vi "AddMenberToRankingList.vi"(2 "Arr引用句柄":refnum<vi>, 3 "玩家信息":T1, 4 "File Path Control":path) -> ()   [LabVIEW 2019]
uses:
  ctl/InfoOfPlayer.ctl
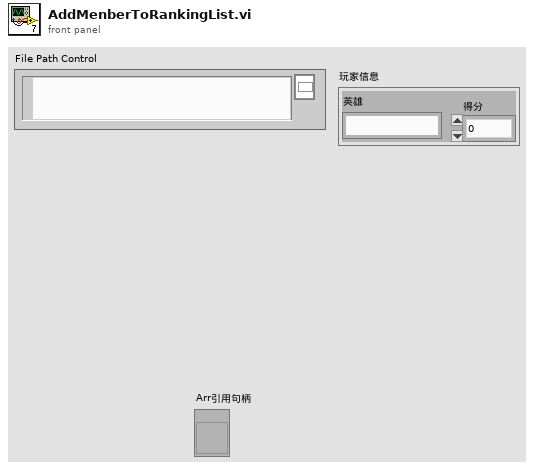
[diagram p1: front panel]
types:
  T1 = typedef "InfoOfPlayer.ctl" = cluster{"得分":i32, "英雄":string}
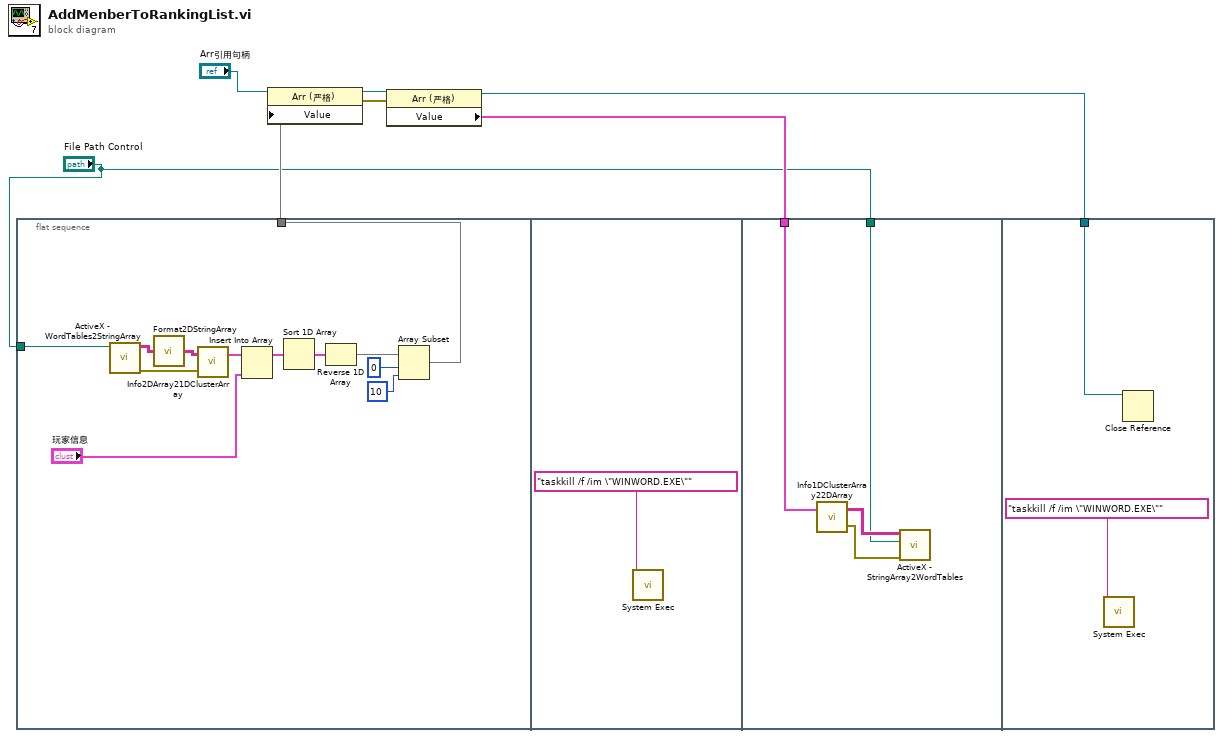
[diagram p0: block diagram]
diagram:
  n1 = flat-sequence {
    tunnel: "File Path Control" -> [w10]
    tunnel: [w8] -> w6
    tunnel: w3 -> [w22]
    tunnel: "File Path Control" -> [w21]
    tunnel: w1 -> [w25]
    frame #0 {
      n2 = call "ActiveX - WordTables2StringArray.vi"("File Path Control"=w10) -> ("Error Out"=w19:errorcluster, "Array"=w11:string[][])  [unwired: 7 in, 2 out]
      n3 = call "Format2DStringArray.vi"("待格式化2D数组"=w11) -> ("格式化2D数组"=w12:string[][])
      n4 = call "Info2DArray21DClusterArray.vi"("error in (no error)"=w19, "2DStringArray"=w12) -> ("1DClusterArray"=w18:T1[])  [unwired: 1 out]
      n5 = Insert Into Array(array=w18, new element="玩家信息") -> (w17:T1[])  [unwired: 1 in]
      n6 = Sort 1D Array(array=w17) -> (sorted array=w14:T1[])
      n7 = Reverse 1D Array(array=w14) -> (reversed array=w13:T1[])
      n8 = Array Subset(array=w13, index=0 ("索引"), length=10 ("长度")) -> (w8:T1[])
    }
    frame #1 {
      n9 = call <vilib>:"System Exec.vi"("command line"="taskkill /f /im \"WINWORD.EXE\"") -> ()  [unwired: 7 in, 4 out]
    }
    frame #2 {
      n10 = call "Info1DClusterArray22DArray.vi"("1D ClusterArray"=w22) -> ("error out"=w24:errorcluster, "2D StringArray"=w23:string[][])  [unwired: 1 in]
      n11 = call "ActiveX - StringArray2WordTables.vi"("error in (no error)"=w24, "文件存储路径"=w21, "文本数组"=w23) -> ()  [unwired: 8 in, 1 out]
    }
    frame #3 {
      n12 = call <vilib>:"System Exec.vi"("command line"="taskkill /f /im \"WINWORD.EXE\"") -> ()  [unwired: 7 in, 4 out]
      n13 = Close Reference(reference=w25) -> ()  [unwired: 1 in, 1 out]
    }
  }
  n14 = property class="Arr (严格)"(reference="Arr引用句柄", "Value"=w6) -> (reference out=w5:refnum<vi>, error out=w4:errorcluster)  [unwired: 1 in]
  n15 = property class="Arr (严格)"(reference=w5, error in=w4) -> (reference out=w1:refnum<vi>, "Value"=w3:T1[])  [unwired: 1 out]
